vi "CloseGen.vi"(8 "error in (no error)":errorcluster, 11 "Instrument Handle":refnum<k15>) -> (0 "error out":errorcluster)   [LabVIEW 2020]
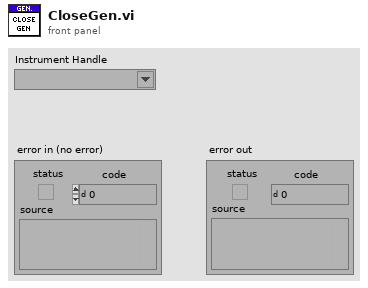
[diagram p1: front panel]
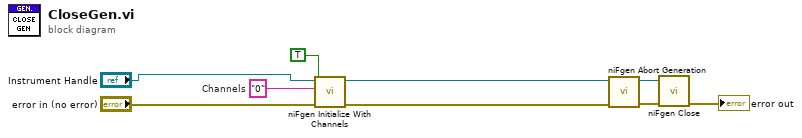
[diagram p0: block diagram]
diagram:
  w6 = "0"  # Channels
  n1 = call <instrlib>:"niFgen Initialize With Channels.vi"("error in (no error)"="error in (no error)", "Reset Device (default: True)"=TRUE, "Channel Name"=w6, "Resource Name"="Instrument Handle") -> ("error out"=w3:errorcluster, "Instrument Handle Out"=w4:refnum<k15>)  [unwired: 6 in]
  n2 = call <instrlib>:"niFgen Abort Generation.vi"("error in (no error)"=w3, "Instrument Handle"=w4) -> ("error out"=w8:errorcluster, "Instrument Handle Out"=w9:refnum<k15>)  [unwired: 8 in]
  n3 = call <instrlib>:"niFgen Close.vi"("error in (no error)"=w8, "Instrument Handle"=w9) -> ("error out"=→"error out":errorcluster)  [unwired: 9 in]
